vi "Stage_Independent.vi"() -> ()   [LabVIEW 2020]
uses:
  Stage/subvi/XImc Example 1 CS.ctl
  Stage/libximc.lvlib
  Stage/Sync_outFlags.ctl
  Stage/Sync_inFlags.ctl
  Stage/StageOptions.ctl
panel:
  in  "SyncOutPeriod":u32
  out "uCurPosition 2":i32
  out "CurPosition 2":i32
  out "uCurPosition":i32
  out "CurPosition":i32
  out "Serial nos.":u32[](array[numeric])
  out "Ids":i32[](array[numeric])
  out "Names":string[](array[string])
  in  "Controller 3":u16(ring) items=["xi-com:\\\\.\\COM4"]
  in  "Controller 2":u16(ring) items=["xi-com:\\\\.\\COM4"]
  out "Cur pos 1":dbl format="%#.2f"
  out "Cur pos 2":dbl format="%#.2f"
  out "Cur pos 3":dbl format="%#.2f"
  out "s/n 1":u32
  out "s/n 3":u32
  out "s/n 2":u32
  in  "Find controllers":bool
  in  "Controller 1":u16(ring) items=["xi-com:\\\\.\\COM4"]
  in  "Stop motion":bool
  in  "Destination 1":i32
  in  "Start move":bool
  in  "Destination 2":i32
  in  "Destination 3":i32
  in  "Destination 4":i32
  in  "Destination 5":i32
  in  "Destination 6":i32
  in  "Close application":bool
  in  "Start shift":bool
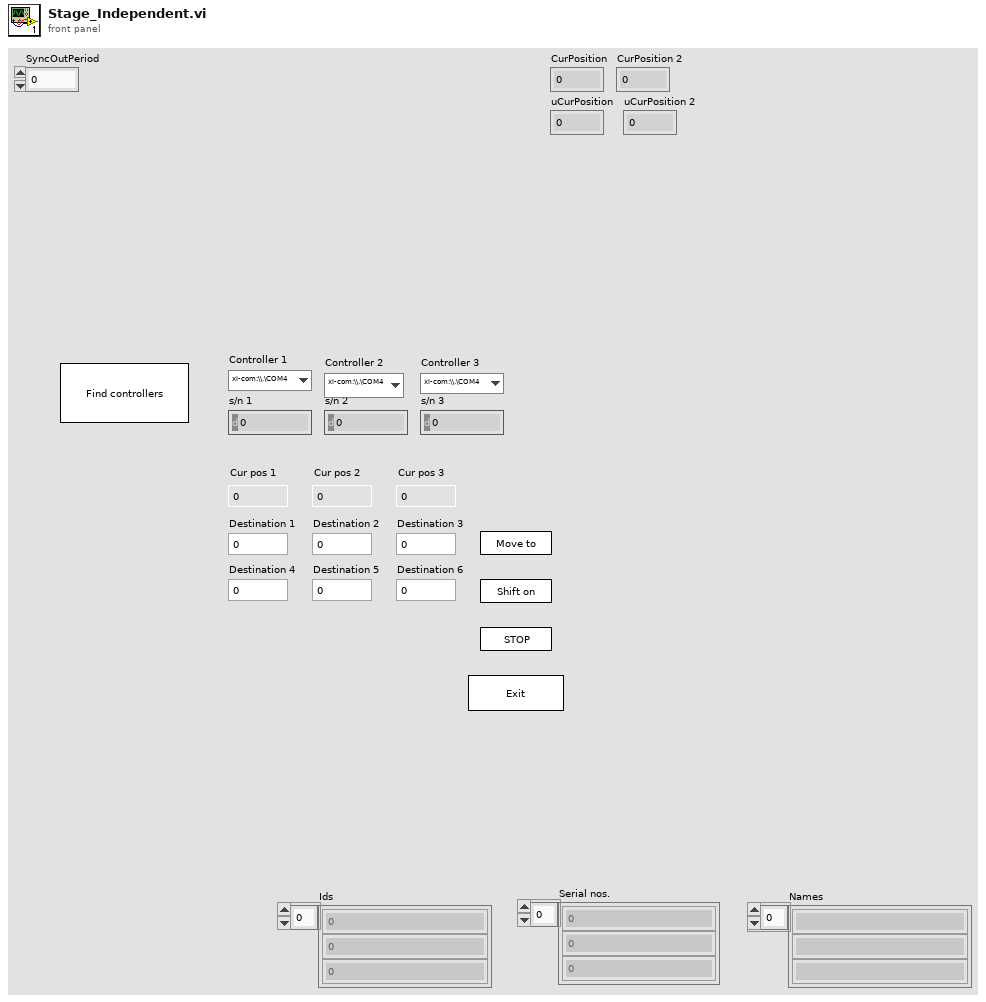
[diagram p1: front panel]
types:
  T1 = typedef "StageOptions.ctl" = enum16{"FindDevices", "Set Trig Settings", "Idle", "Get Status", "MoveX - Right", "MoveX - Left", "MoveY - Up", "MoveY - Down"}
  T2 = typedef "XImc Example 1 CS.ctl" = enum16{"Initialize_App", "Idle", "Find_Controllers", "Initialize_Controller", "Set_Parameters", "Get_Status", "Start_Motion", "Move_Relative", "Stop_Motion", "ZEROCOMM", "HOME", "LEFT", "RIGT", "SSTP", "Close_Controller", "Error_Handler", "Close_App", "Get_Move_Settings", "Set_Move_Settings"}
  T3 = cluster{"Number of controllers":i32, "Controllers' names":string[], "variant":variant, "quit":bool, "IDs":i32[]}
  T4 = cluster{"Destination 4":i32, "Destination 5":i32, "Destination 6":i32}
  T5 = cluster{"Destination 1":i32, "Destination 2":i32, "Destination 3":i32}
  T6 = cluster{"MoveSts":u32, "MvCmdSts":u32, "PWRSts":u32, "EncSts":u32, "WindSts":u32, "CurPosition":i32, "uCurPosition":i32, "@dummy control@":i8, "@dummy control@":i8, "@dummy control@":i8, "@dummy control@":i8, "EncPosition":i64, "CurSpeed":i32, "uCurSpeed":i32, "Ipwr":i32, "Upwr":i32, "Iusb":i32, "Uusb":i32, "CurT":i32, "Flags":u32, "GPIOFlags":u32, "CmdBufFreeSpace":u32}
  T7 = typedef "Sync_outFlags.ctl" = cluster{"Enabled":bool, "state":bool, "invert":bool, "in_steps":bool, "on_start":bool, "on_stop":bool, "on_period":bool}
  T8 = cluster{"SyncOutFlags":u32, "SyncOutPulseSteps":u32, "SyncOutPeriod":u32, "Accuracy":u32, "uAccuracy":u32}
  T9 = typedef "Sync_inFlags.ctl" = cluster{"Enabled":bool, "invert":bool, "go_to_position":bool}
  T10 = cluster{"SyncInFlags":u32, "ClutterTime":u32, "Position":i32, "uPosition":i32, "Speed":u32, "uSpeed":u32}
  T11 = cluster{"SyncOutFlags":u32, "SyncOutPulseSteps":u32, "SyncOutPeriod":u32, "Accuracy":u32, "uAccuracy":u32}[]
  T12 = cluster{"SyncInFlags":u32, "ClutterTime":u32, "Position":i32, "uPosition":i32, "Speed":u32, "uSpeed":u32}[]
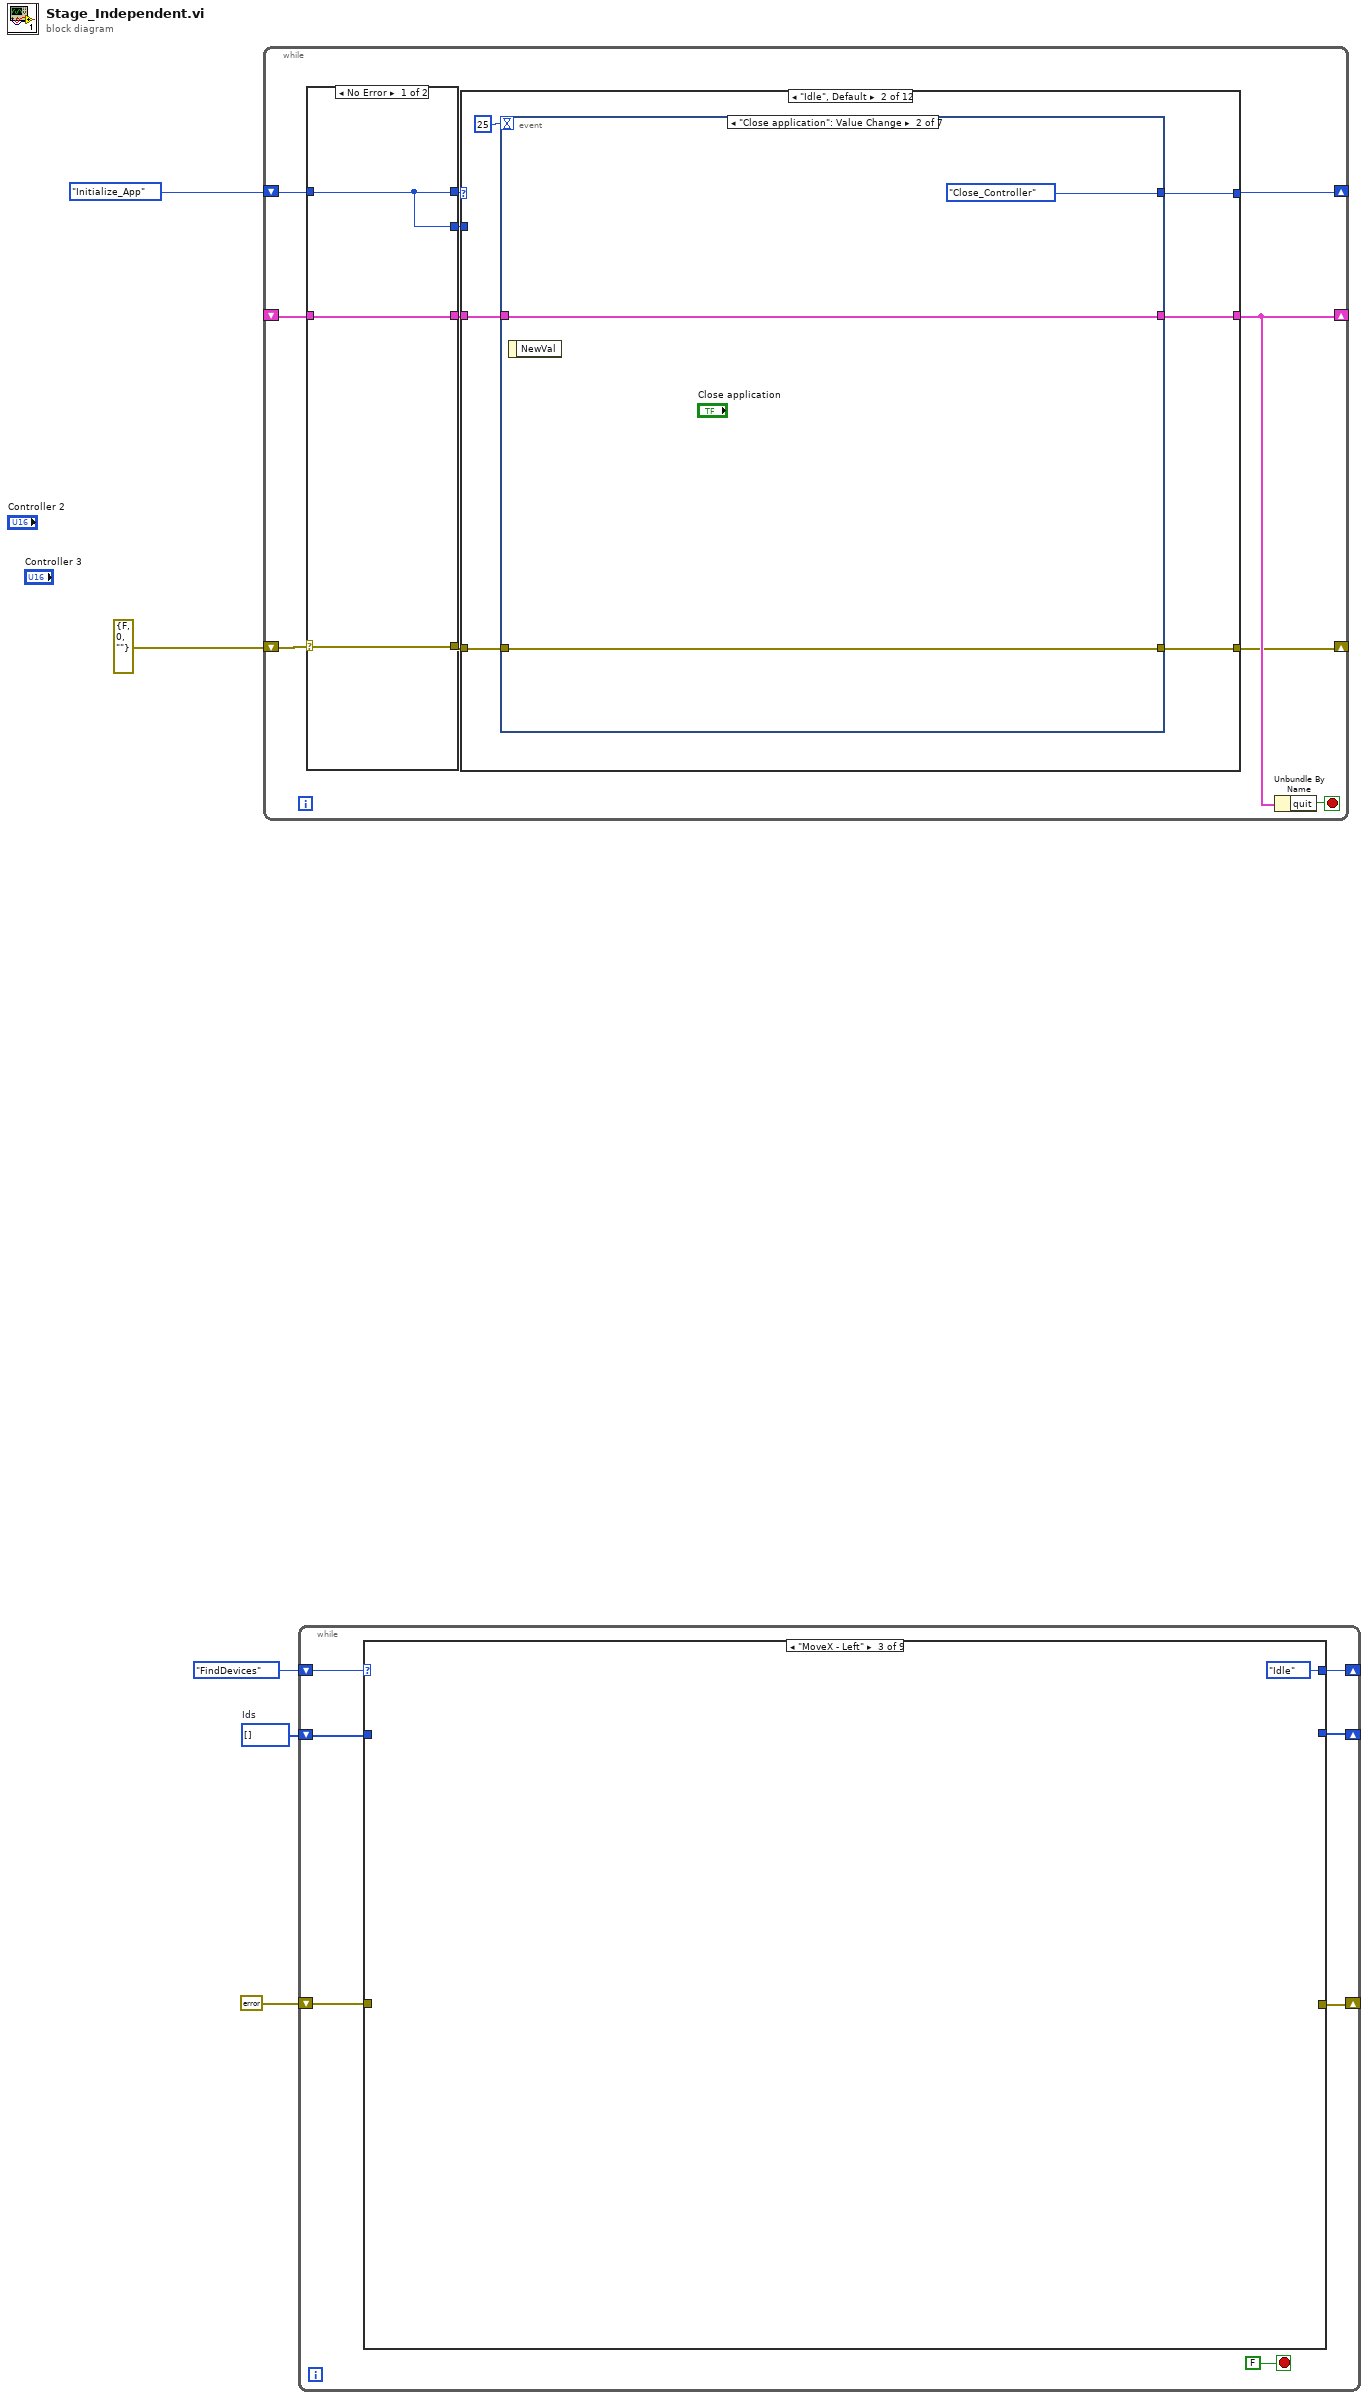
[diagram p0: block diagram]
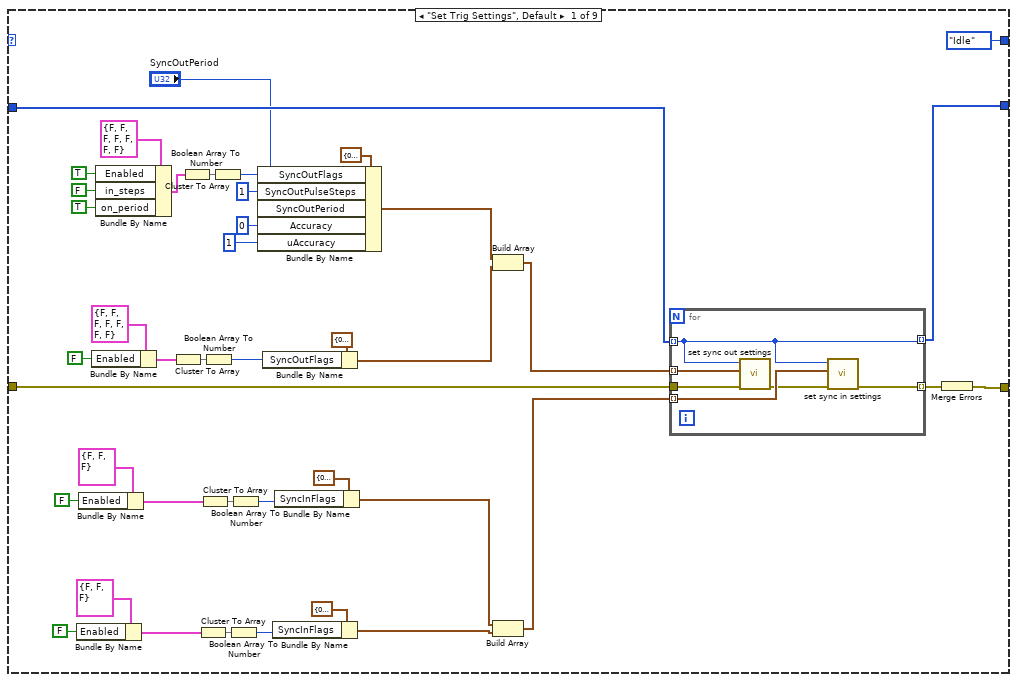
[diagram p2: hidden frame]
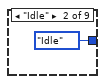
[diagram p3: hidden frame]
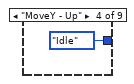
[diagram p4: hidden frame]
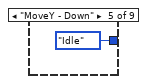
[diagram p5: hidden frame]
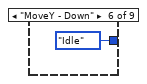
[diagram p6: hidden frame]
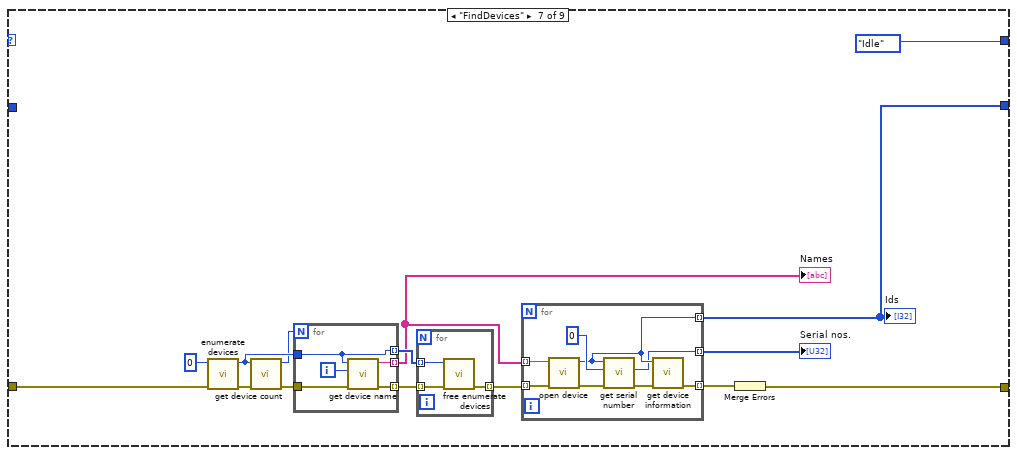
[diagram p7: hidden frame]
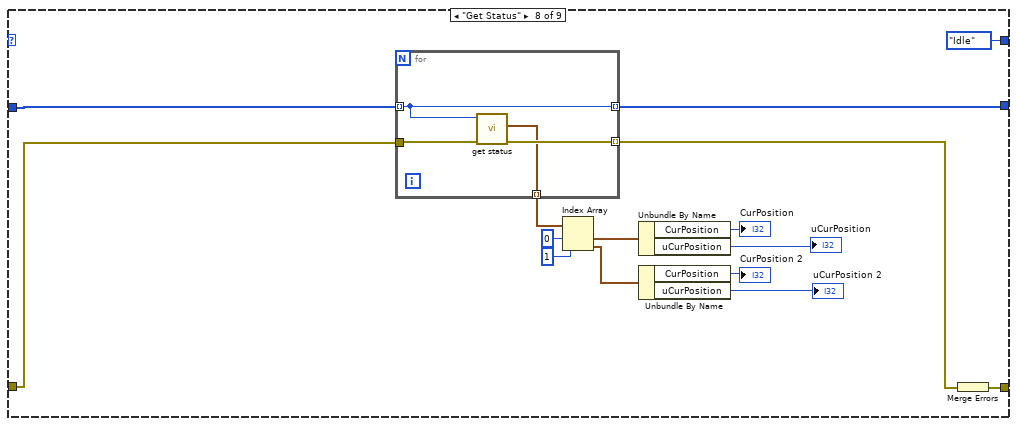
[diagram p8: hidden frame]
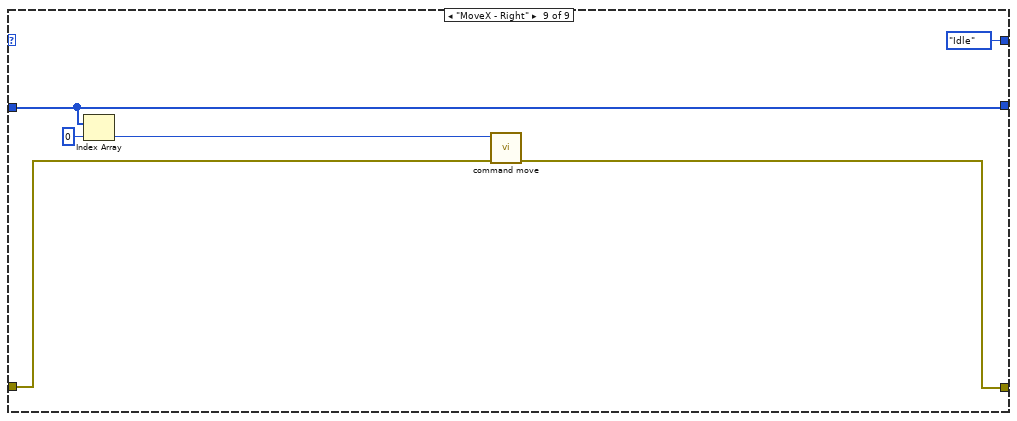
[diagram p9: hidden frame]
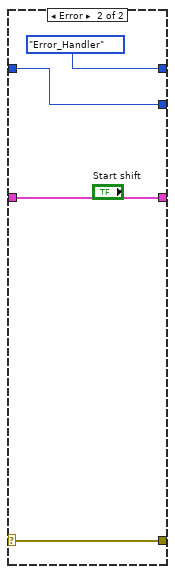
[diagram p10: hidden frame]
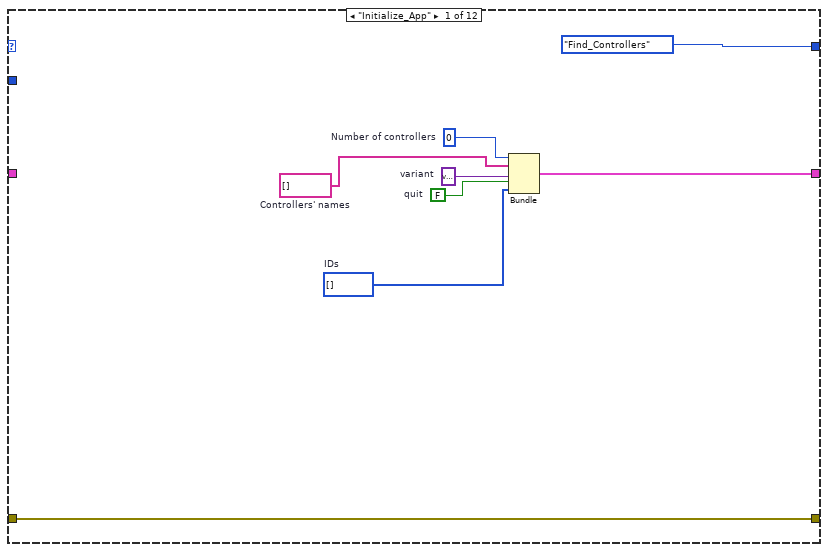
[diagram p11: hidden frame]
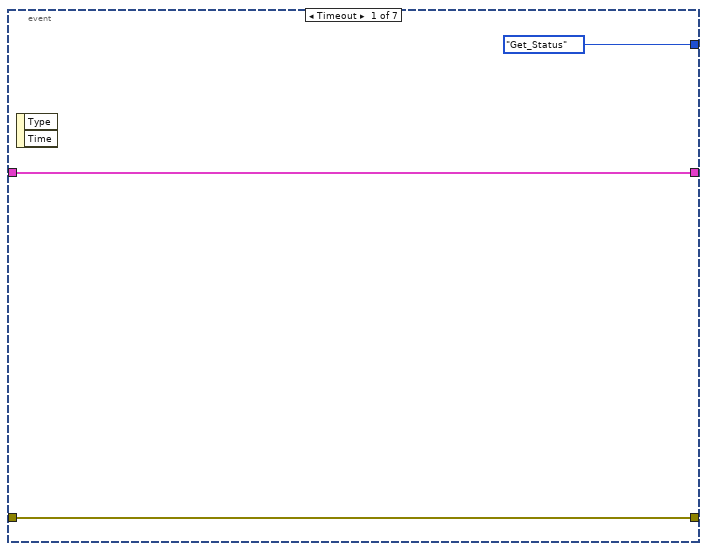
[diagram p12: hidden frame]
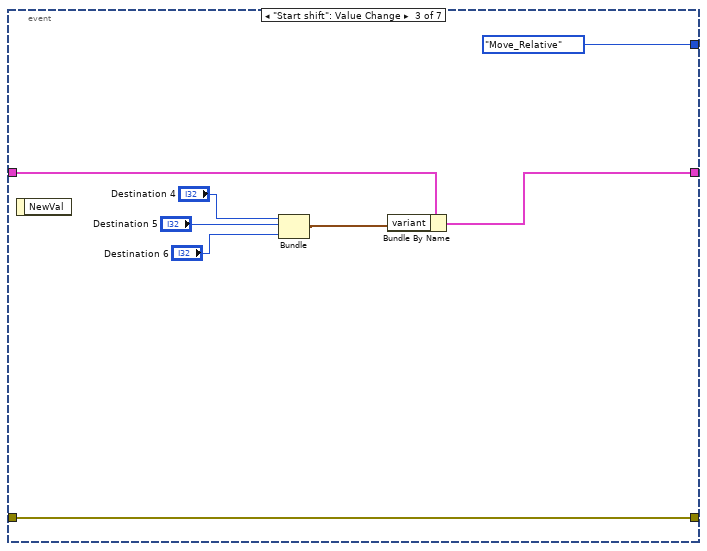
[diagram p13: hidden frame]
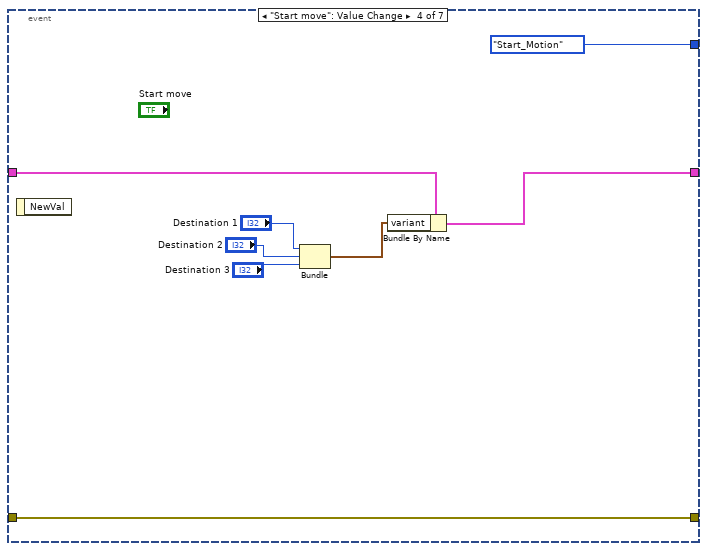
[diagram p14: hidden frame]
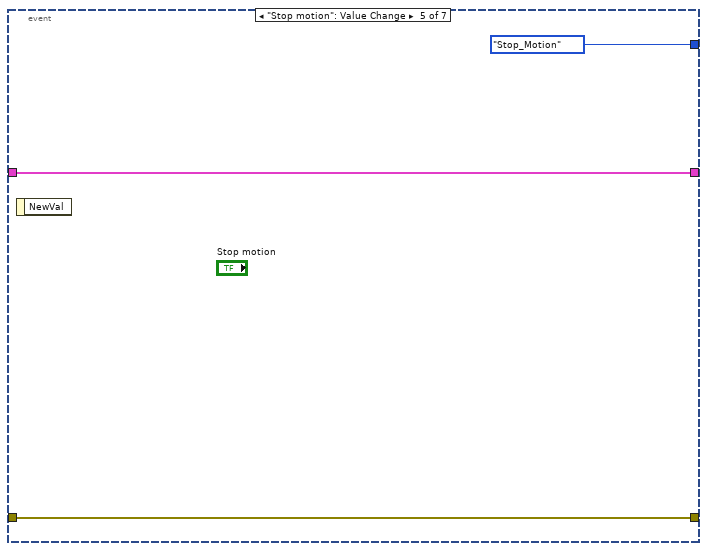
[diagram p15: hidden frame]
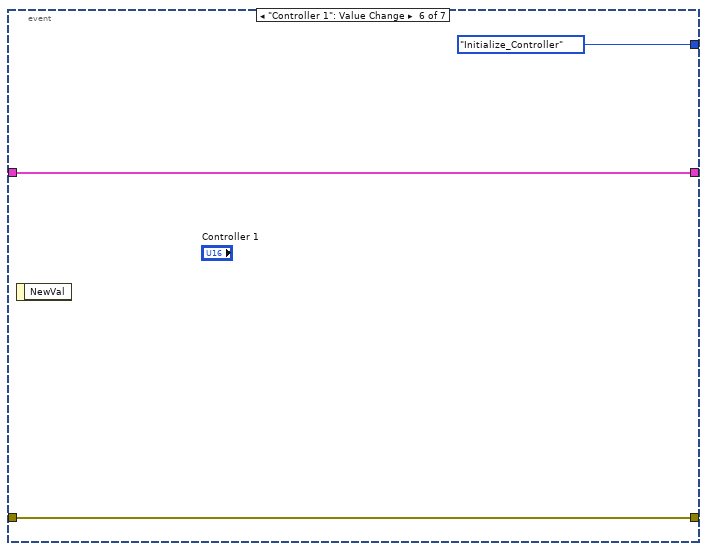
[diagram p16: hidden frame]
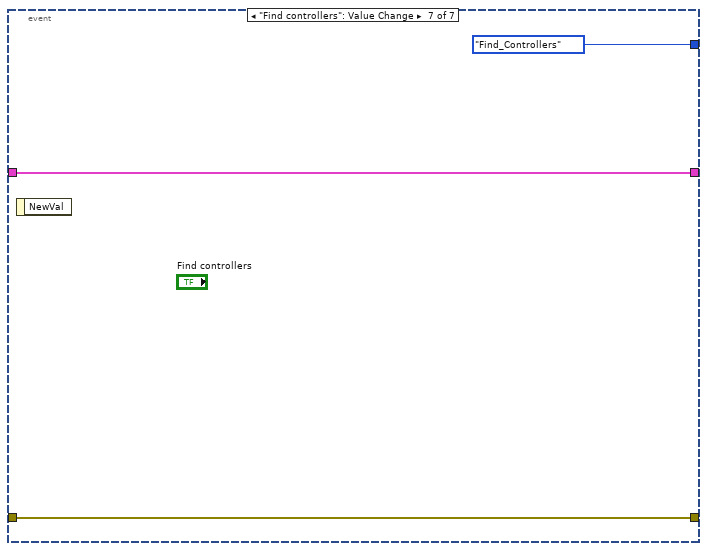
[diagram p17: hidden frame]
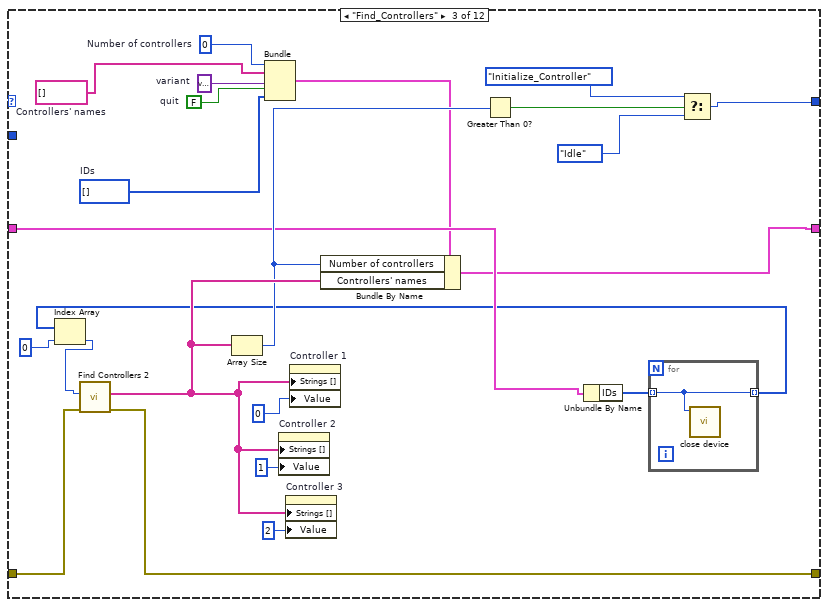
[diagram p18: hidden frame]
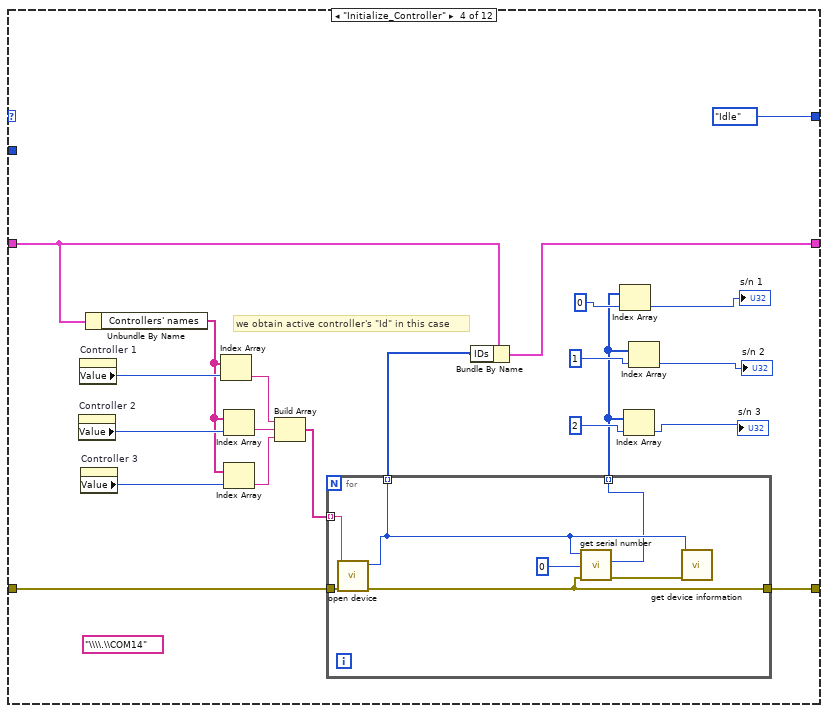
[diagram p19: hidden frame]
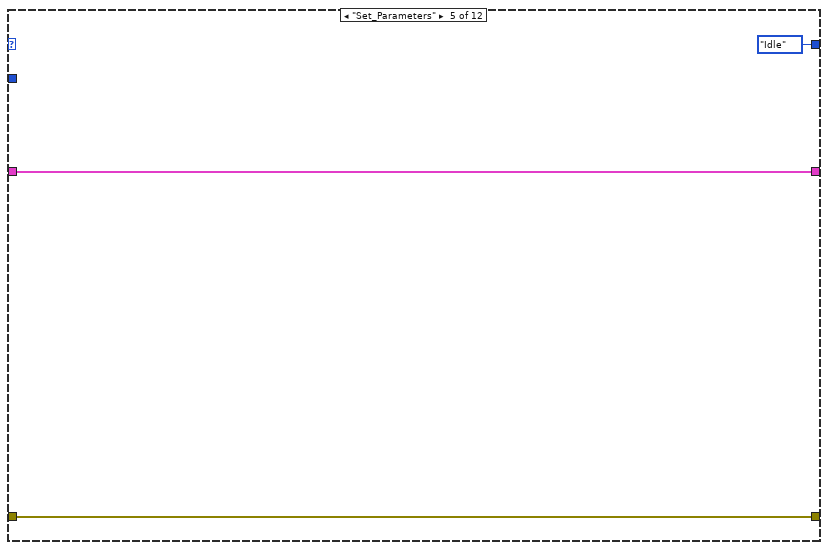
[diagram p20: hidden frame]
diagram:
  w2 = i32[] []  # Ids
  n1 = while {
    shift-right: [w16] -> _
    shift-left: XImc_Example_1_CS."Initialize_App" ("Case") -> [w10]
    shift-right: [w15] -> _
    shift-left: _ -> [w12]
    shift-right: [w7] -> _
    shift-left: errorcluster {"status"=FALSE, "code"=0, "source"=""} ("error in (no error)") -> [w14]
    stop <- w6 stop-if-true
    n2 = case shown="No Error" w14 {
      selector: w14 -> [w19 w22]
      tunnel: [w19 w22] -> w13
      tunnel: w12 -> [w18 w20]
      tunnel: [w18 w20] -> w11
      tunnel: w10 -> [w17 w21]
      tunnel: [w17 XImc_Example_1_CS."Error_Handler" ("Case")] -> w9
      tunnel: [w17 w21] -> w8
      frame No Error {
      }
      frame Error {
      }
    }
    n3 = case shown="\"Idle\", Default" w9 {
      tunnel: [XImc_Example_1_CS."Find_Controllers" ("Case") w35 w89 XImc_Example_1_CS."Idle" ("Case") XImc_Example_1_CS."Idle" ("Case") XImc_Example_1_CS."Idle" ("Case") XImc_Example_1_CS."Idle" ("Case") XImc_Example_1_CS."Idle" ("Case") XImc_Example_1_CS."Idle" ("Case") XImc_Example_1_CS."Close_App" ("Case") w195 XImc_Example_1_CS."Idle" ("Case")] -> w16
      tunnel: [w24 w34 w74 w110 w122 w134 w151 w158 w173 w180 w194 w197] -> w15
      tunnel: w13 -> [w28 w37 w70 w111 w121 w136 w150 w160 w172 w179 w193 w200]
      tunnel: w11 -> [_ w33 w81 w105 w122 w134 w151 w158 w173 w180 w194 w198]
      tunnel: w8 -> [_ _ _ _ _ _ _ _ _ _ w195 _]
      tunnel: [w28 w32 w69 w109 w121 w135 w149 w159 w170 w181 w192 w200] -> w7
      frame "Initialize_App" {
        w25 = i32[] []  # IDs
        w26 = string[] []  # Controllers' names
        w27 = 0  # Number of controllers
        w29 = FALSE  # quit
        w30 = variant  # variant
        n4 = Bundle("Number of controllers"=w27, "Controllers' names"=w26, "variant"=w30, "quit"=w29, "IDs"=w25) -> (w24:T3)  [unwired: 1 in]
      }
      frame "Idle", Default {
        n5 = event shown="[1] \"Close application\": Value Change" {
          selector: _ -> [_ _ _ _ _ _ _]
          dyn-events: _ -> [_ _ _ _ _ _ _]
          timeout: 25 -> [_ _ _ _ _ _ _]
          tunnel: w37 -> [w38 w41 w50 w58 w61 w64 w66]
          tunnel: [XImc_Example_1_CS."Get_Status" ("Case") XImc_Example_1_CS."Close_Controller" ("Case") XImc_Example_1_CS."Move_Relative" ("Case") XImc_Example_1_CS."Start_Motion" ("Case") XImc_Example_1_CS."Stop_Motion" ("Case") XImc_Example_1_CS."Initialize_Controller" ("Case") XImc_Example_1_CS."Find_Controllers" ("Case")] -> w35
          tunnel: [w39 w42 w48 w56 w60 w63 w67] -> w34
          tunnel: w33 -> [w39 w42 w49 w57 w60 w63 w67]
          tunnel: [w38 w41 w50 w58 w61 w64 w66] -> w32
          event Timeout {
            n6 = event-data() -> ()  [unwired: 1 in, 2 out]
          }
          event "Close application": Value Change {
            n7 = event-data() -> ()  [unwired: 1 in, 1 out]
          }
          event "Start shift": Value Change {
            n8 = event-data() -> ()  [unwired: 1 in, 1 out]
            n9 = Bundle("Destination 4"="Destination 4", "Destination 5"="Destination 5", "Destination 6"="Destination 6") -> (w47:T4)  [unwired: 1 in]
            n10 = Bundle By Name(cluster=w49, "variant"=w47) -> (w48:T3)
          }
          event "Start move": Value Change {
            n11 = event-data() -> ()  [unwired: 1 in, 1 out]
            n12 = Bundle("Destination 1"="Destination 1", "Destination 2"="Destination 2", "Destination 3"="Destination 3") -> (w52:T5)  [unwired: 1 in]
            n13 = Bundle By Name(cluster=w57, "variant"=w52) -> (w56:T3)
          }
          event "Stop motion": Value Change {
            n14 = event-data() -> ()  [unwired: 1 in, 1 out]
          }
          event "Controller 1": Value Change {
            n15 = event-data() -> ()  [unwired: 1 in, 1 out]
          }
          event "Find controllers": Value Change {
            n16 = event-data() -> ()  [unwired: 1 in, 1 out]
          }
        }
      }
      frame "Find_Controllers" {
        w76 = i32[] []  # IDs
        w77 = string[] []  # Controllers' names
        w78 = 0  # Number of controllers
        w79 = FALSE  # quit
        w80 = variant  # variant
        n17 = Bundle("Number of controllers"=w78, "Controllers' names"=w77, "variant"=w80, "quit"=w79, "IDs"=w76) -> (w75:T3)  [unwired: 1 in]
        n18 = Unbundle By Name(w81) -> ("IDs"=w82:i32[])
        n19 = for {
          tunnel: w82 -> [w92] mode=indexing
          tunnel: [w92] -> w73 mode=indexing
          n20 = call "close device.vi"("id"=w92) -> ()  [unwired: 8 in, 3 out]
        }
        n21 = Index Array(array=w73, index=0) -> (element=w72:i32)
        n22 = call "Find Controllers 2.vi"("error in (no error)"=w70, "Numeric"=w72) -> ("error out"=w69:errorcluster, "Names"=w84:string[])  [unwired: 8 in]
        n23 = Array Size(array=w84) -> (size(s)=w83:i32)
        n24 = property on="Controller 2" class="Ring (strict)"("Strings []"=w84, "Value"=1) -> ()  [unwired: 2 in, 2 out]
        n25 = property on="Controller 3" class="Ring (strict)"("Strings []"=w84, "Value"=2) -> ()  [unwired: 2 in, 2 out]
        n26 = property on="Controller 1" class="Ring (strict)"("Strings []"=w84, "Value"=0) -> ()  [unwired: 2 in, 2 out]
        n27 = Bundle By Name(cluster=w75, "Number of controllers"=w83, "Controllers' names"=w84) -> (w74:T3)
        n28 = Greater Than 0?(x=w83) -> (x > 0?=w91:bool)
        n29 = Select(t=XImc_Example_1_CS."Initialize_Controller", s=w91, f=XImc_Example_1_CS."Idle" ("Case")) -> (s? t:f=w89:T2)
      }
      frame "Initialize_Controller" {
        (unwired) "\\\\.\\COM14" ("name")
        # "we obtain active controller's \"Id\" in this case"
        n30 = property on="Controller 2" class="Ring (strict)"() -> ("Value"=w107:u16)  [unwired: 2 in, 2 out]
        n31 = property on="Controller 1" class="Ring (strict)"() -> ("Value"=w112:u16)  [unwired: 2 in, 2 out]
        n32 = property on="Controller 3" class="Ring (strict)"() -> ("Value"=w106:u16)  [unwired: 2 in, 2 out]
        n33 = Unbundle By Name(w105) -> ("Controllers' names"=w100:string[])
        n34 = Index Array(array=w100, index=w112) -> (element=w102:string)
        n35 = Index Array(array=w100, index=w107) -> (element=w103:string)
        n36 = Index Array(array=w100, index=w106) -> (element=w104:string)
        n37 = Build Array(w102, w103, w104) -> (w101:string[])
        n38 = for {
          tunnel: w111 -> [w120]
          tunnel: [w116] -> w109
          tunnel: [w117] -> w108 mode=indexing
          tunnel: w101 -> [w115] mode=indexing
          tunnel: [w114] -> w96 mode=indexing
          n39 = call "open device.vi"("error in (no error)"=w120, "uri"=w115) -> ("error out"=w116:errorcluster, "function return"=w117:i32)  [unwired: 8 in]
          n40 = call "get serial number.vi"("error in (no error)"=w116, "SerialNumber"=u32 0 ("serial"), "id"=w117) -> ("error out"=w118:errorcluster, "SerialNumber out"=w114:u32)  [unwired: 6 in, 1 out]
          n41 = call "get device information.vi"("error in (no error)"=w118, "id"=w117) -> ()  [unwired: 7 in, 3 out]
        }
        n42 = Bundle By Name(cluster=w105, "IDs"=w108) -> (w110:T3)
        n43 = Index Array(array=w96, index=u32 0 ("serial")) -> (element=→"s/n 1":u32)
        n44 = Index Array(array=w96, index=u32 2 ("serial")) -> (element=→"s/n 3":u32)
        n45 = Index Array(array=w96, index=u32 1 ("serial")) -> (element=→"s/n 2":u32)
      }
      frame "Set_Parameters" {
      }
      frame "Get_Status" {
        n46 = Unbundle By Name(w134) -> ("IDs"=w133:i32[])
        n47 = for {
          tunnel: w136 -> [w143]
          tunnel: [w142] -> w135
          tunnel: [w141] -> w131 mode=indexing
          tunnel: w133 -> [w138] mode=indexing
          tunnel: [w140] -> w132 mode=indexing
          n48 = call "get status.vi"("error in (no error)"=w143, "id"=w138) -> ("error out"=w142:errorcluster, "status out"=w139:T6, "function return"=w140:i32)  [unwired: 7 in]
          n49 = Unbundle By Name(w139) -> ("CurPosition"=w141:i32)
        }
        n50 = Greater Or Equal To 0?(x=w132) -> (x >= 0?=w124:bool[])
        n51 = And Array Elements(Boolean array=w124) -> ()  [unwired: 1 out]
        n52 = Index Array(array=w131, index #1=0 ("index"), index #2=1 ("index"), index #3=2 ("index")) -> (element #1=→"Cur pos 1":i32, element #2=→"Cur pos 2":i32, element #3=→"Cur pos 3":i32)
      }
      frame "Start_Motion" {
        n53 = Unbundle By Name(w151) -> ("IDs"=w147:i32[], "variant"=w144:variant)
        n54 = Variant To Data(type=cluster{u32, u32, u32} {0, 0, 0}, Variant=w144) -> (data=w148:cluster{u32, u32, u32})  [unwired: 1 in, 1 out]
        n55 = Cluster To Array(cluster=w148) -> (array=w145:u32[])
        n56 = for {
          tunnel: w150 -> [w156]
          tunnel: [w155] -> w149
          tunnel: w145 -> [w154] mode=indexing
          tunnel: w147 -> [w153] mode=indexing
          n57 = call "command move.vi"("error in (no error)"=w156, "Position"=w154, "id"=w153) -> ("error out"=w155:errorcluster)  [unwired: 7 in, 1 out]
        }
      }
      frame "Move_Relative" {
        n58 = Unbundle By Name(w158) -> ("IDs"=w163:i32[], "variant"=w157:variant)
        n59 = Variant To Data(type=cluster{u32, u32, u32} {0, 0, 0}, Variant=w157) -> (data=w164:cluster{u32, u32, u32})  [unwired: 1 in, 1 out]
        n60 = Cluster To Array(cluster=w164) -> (array=w161:u32[])
        n61 = for {
          tunnel: w160 -> [w168]
          tunnel: [w167] -> w159
          tunnel: w161 -> [w169] mode=indexing
          tunnel: w163 -> [w166] mode=indexing
          n62 = call "command movr.vi"("error in (no error)"=w168, "DeltaPosition"=w169, "id"=w166) -> ("error out"=w167:errorcluster)  [unwired: 7 in, 1 out]
        }
      }
      frame "Stop_Motion" {
        n63 = Unbundle By Name(w173) -> ("IDs"=w171:i32[])
        n64 = for {
          tunnel: w172 -> [w177]
          tunnel: w171 -> [w175] mode=indexing
          tunnel: [w176] -> w170
          n65 = call "command stop.vi"("error in (no error)"=w177, "id"=w175) -> ("error out"=w176:errorcluster)  [unwired: 8 in, 1 out]
        }
      }
      frame "Close_Controller" {
        n66 = Unbundle By Name(w180) -> ("IDs"=w178:i32[])
        n67 = for {
          tunnel: [w186] -> w182
          tunnel: w179 -> [w185]
          tunnel: w178 -> [w184] mode=indexing
          n68 = call "close device.vi"("error in (no error)"=w185, "id"=w184) -> ("error out"=w186:errorcluster)  [unwired: 7 in, 2 out]
        }
        n69 = disable-structure shown="Disabled" {
          disable-tunnel: w182 -> [w191 _]
          disable-tunnel: [w190 _] -> w181
          disable-tunnel: w180 -> [w189 _]
          frame Disabled {
            n70 = Unbundle By Name(w189) -> ("Number of controllers"=w188:i32, "Controllers' names"=w187:string[])
            n71 = call "free enumerate devices.vi"("error in (no error)"=w191, 10:w187, "device_enumeration"=w188) -> ("error out"=w190:errorcluster)  [unwired: 7 in, 1 out]
          }
          frame Enabled {
          }
        }
      }
      frame "Error_Handler" {
        # "here we return to the last case before error occured"
        n72 = call <vilib>:"Clear Errors.vi"("error in (no error)"=w193) -> ("error out"=w192:errorcluster)  [unwired: 5 in, 1 out]
      }
      frame "Close_App" {
        n73 = Bundle By Name(cluster=w198, "quit"=TRUE) -> (w197:T3)
      }
    }
    n74 = Unbundle By Name(w15) -> ("quit"=w6:bool)
  }
  n75 = while {
    shift-right: [w205] -> _
    shift-left: errorcluster {"status"=FALSE, "code"=0, "source"=""} ("error in (no error)") -> [w206]
    shift-right: [w204] -> _
    shift-left: w2 -> [w203]
    shift-right: [w201] -> _
    shift-left: StageOptions."FindDevices" -> [w202]
    stop <- FALSE stop-if-true
    n76 = case shown="\"MoveX - Left\"" w202 {
      tunnel: w206 -> [w237 _ _ _ _ _ w265 w304 w313]
      tunnel: [w236 _ _ _ _ _ w263 w303 w312] -> w205
      tunnel: [StageOptions."Idle" StageOptions."Idle" StageOptions."Idle" StageOptions."Idle" StageOptions."Idle" StageOptions."Idle" StageOptions."Idle" StageOptions."Idle" StageOptions."Idle"] -> w201
      tunnel: [w248 _ _ _ _ _ w262 w305 w311] -> w204
      tunnel: w203 -> [w249 _ _ _ _ _ _ w306 w311]
      frame "Set Trig Settings", Default {
        n77 = Bundle By Name(cluster=T9 {"Enabled"=FALSE, "invert"=FALSE, "go_to_position"=FALSE} ("Sync_out Flags"), "Enabled"=FALSE) -> (w226:T9)
        n78 = Bundle By Name(cluster=T9 {"Enabled"=FALSE, "invert"=FALSE, "go_to_position"=FALSE} ("Sync_out Flags"), "Enabled"=FALSE) -> (w242:T9)
        n79 = Bundle By Name(cluster=T7 {"Enabled"=FALSE, "state"=FALSE, "invert"=FALSE, "in_steps"=FALSE, "on_start"=FALSE, "on_stop"=FALSE, "on_period"=FALSE} ("Sync_out Flags"), "Enabled"=FALSE) -> (w220:T7)
        n80 = Bundle By Name(cluster=T7 {"Enabled"=FALSE, "state"=FALSE, "invert"=FALSE, "in_steps"=FALSE, "on_start"=FALSE, "on_stop"=FALSE, "on_period"=FALSE} ("Sync_out Flags"), "Enabled"=TRUE, "in_steps"=FALSE ("state"), "on_period"=TRUE) -> (w247:T7)
        n81 = Cluster To Array(cluster=w220) -> (array=w221:bool[])
        n82 = Cluster To Array(cluster=w247) -> (array=w246:bool[])
        n83 = Cluster To Array(cluster=w226) -> (array=w227:bool[])
        n84 = Cluster To Array(cluster=w242) -> (array=w241:bool[])
        n85 = Boolean Array To Number(Boolean array=w221) -> (number=w222:u32)
        n86 = Boolean Array To Number(Boolean array=w246) -> (number=w245:u32)
        n87 = Boolean Array To Number(Boolean array=w227) -> (number=w228:u32)
        n88 = Boolean Array To Number(Boolean array=w241) -> (number=w240:u32)
        n89 = Bundle By Name(cluster=T8 {"SyncOutFlags"=0, "SyncOutPulseSteps"=0, "SyncOutPeriod"=0, "Accuracy"=0, "uAccuracy"=0} ("sync_out_settings"), "SyncOutFlags"=w245, "SyncOutPulseSteps"=u32 1, "SyncOutPeriod"="SyncOutPeriod", "Accuracy"=u32 0, "uAccuracy"=u32 1) -> (w234:T8)
        n90 = Bundle By Name(cluster=T8 {"SyncOutFlags"=0, "SyncOutPulseSteps"=0, "SyncOutPeriod"=0, "Accuracy"=0, "uAccuracy"=0} ("sync_out_settings"), "SyncOutFlags"=w222) -> (w219:T8)
        n91 = Bundle By Name(cluster=T10 {"SyncInFlags"=0, "ClutterTime"=0, "Position"=0, "uPosition"=0, "Speed"=0, "uSpeed"=0} ("sync_in_settings"), "SyncInFlags"=w228) -> (w225:T10)
        n92 = Bundle By Name(cluster=T10 {"SyncInFlags"=0, "ClutterTime"=0, "Position"=0, "uPosition"=0, "Speed"=0, "uSpeed"=0} ("sync_in_settings"), "SyncInFlags"=w240) -> (w232:T10)
        n93 = Build Array(w234, w219) -> (w233:T11)
        n94 = Build Array(w232, w225) -> (w231:T12)
        n95 = for {
          tunnel: w249 -> [w253] mode=indexing
          tunnel: [w253] -> w248 mode=indexing
          tunnel: w233 -> [w255] mode=indexing
          tunnel: w231 -> [w254] mode=indexing
          tunnel: w237 -> [w251]
          tunnel: [w250] -> w235 mode=indexing
          n96 = call "set sync out settings.vi"("error in (no error)"=w251, "sync_out_settings"=w255, "id"=w253) -> ("error out"=w252:errorcluster)  [unwired: 7 in, 1 out]
          n97 = call "set sync in settings.vi"("error in (no error)"=w252, "sync_in_settings"=w254, "id"=w253) -> ("error out"=w250:errorcluster)  [unwired: 7 in, 1 out]
        }
        n98 = Merge Errors(w235) -> (w236:errorcluster)
      }
      frame "Idle" {
      }
      frame "MoveX - Left" {
      }
      frame "MoveY - Up" {
      }
      frame "MoveY - Down" {
      }
      frame "MoveY - Down" {
      }
      frame "FindDevices" {
        n99 = call "enumerate devices.vi"("error in (no error)"=w265, "enumerate_flags"=0 ("probe_devices")) -> ("error out"=w269:errorcluster, "function return"=w270:u32)  [unwired: 8 in]
        n100 = call "get device count.vi"("error in (no error)"=w269, "device_enumeration"=w270) -> ("error out"=w268:errorcluster, "function return"=w267:i32)  [unwired: 8 in]
        n101 = for {
          N: w267 -> [_]
          tunnel: [w291] -> w274 mode=indexing
          tunnel: [w290] -> w271 mode=indexing
          tunnel: w270 -> [w287]
          tunnel: w268 -> [w288]
          tunnel: [w287] -> w273 mode=indexing
          i -> [w289]
          n102 = call "get device name.vi"("error in (no error)"=w288, "device_index"=w289, "device_enumeration"=w287) -> ("error out"=w291:errorcluster, "function return"=w290:string)  [unwired: 7 in]
        }
        "Names" <- w271
        n103 = for {
          tunnel: w273 -> [w278] mode=indexing
          tunnel: w274 -> [w277] mode=indexing
          tunnel: [w276] -> w275 mode=indexing
          n104 = call "free enumerate devices.vi"("error in (no error)"=w277, "device_enumeration"=w278) -> ("error out"=w276:errorcluster)  [unwired: 8 in, 1 out]
        }
        n105 = for {
          tunnel: w275 -> [w286] mode=indexing
          tunnel: [w283] -> w262 mode=indexing
          tunnel: w271 -> [w281] mode=indexing
          tunnel: [w280] -> w272 mode=indexing
          tunnel: [w279] -> w264 mode=indexing
          n106 = call "open device.vi"("error in (no error)"=w286, "uri"=w281) -> ("error out"=w282:errorcluster, "function return"=w283:i32)  [unwired: 8 in]
          n107 = call "get serial number.vi"("error in (no error)"=w282, "SerialNumber"=u32 0 ("serial"), "id"=w283) -> ("error out"=w284:errorcluster, "SerialNumber out"=w280:u32)  [unwired: 6 in, 1 out]
          n108 = call "get device information.vi"("error in (no error)"=w284, "id"=w283) -> ("error out"=w279:errorcluster)  [unwired: 7 in, 2 out]
        }
        "Ids" <- w262
        "Serial nos." <- w272
        n109 = Merge Errors(w264) -> (w263:errorcluster)
      }
      frame "Get Status" {
        n110 = for {
          tunnel: w306 -> [w310] mode=indexing
          tunnel: [w310] -> w305 mode=indexing
          tunnel: w304 -> [w309]
          tunnel: [w308] -> w302 mode=indexing
          tunnel: [w307] -> w301 mode=indexing
          n111 = call "get status.vi"("error in (no error)"=w309, "id"=w310) -> ("error out"=w308:errorcluster, "status out"=w307:T6)  [unwired: 7 in, 1 out]
        }
        n112 = Index Array(array=w301, index #1=0 ("index"), index #2=1 ("index")) -> (element #1=w298:T6, element #2=w297:T6)
        n113 = Unbundle By Name(w298) -> ("CurPosition"=→"CurPosition":i32, "uCurPosition"=→"uCurPosition":i32)
        n114 = Unbundle By Name(w297) -> ("CurPosition"=→"CurPosition 2":i32, "uCurPosition"=→"uCurPosition 2":i32)
        n115 = Merge Errors(w302) -> (w303:errorcluster)
      }
      frame "MoveX - Right" {
        n116 = Index Array(array=w311, index=0) -> (element=w315:i32)
        n117 = call "command move.vi"("error in (no error)"=w313, "id"=w315) -> ("error out"=w312:errorcluster)  [unwired: 8 in, 1 out]
      }
    }
  }
